vi "Pre-Bury Hook.vi"(8 "Error In":errorcluster) -> (0 "Error Out":errorcluster)   [LabVIEW 2018, in "Tests.lvlib" / "Toolkit.lvlib" / "Integration.lvlib"]
uses:
  Integration.lvlib
  Support/Bury Target.vi
  src/Toolkit/Toolkit.lvlib
  <vilib>/addons/_JKI Toolkits/Caraya/classes/Test/Test.lvclass
  Tests.lvlib
  <vilib>/addons/_JKI Toolkits/Caraya/classes/Assert/Assert.lvclass
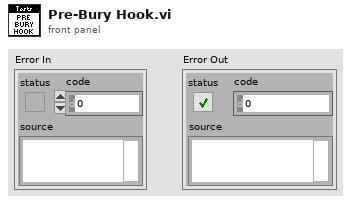
[diagram p1: front panel]
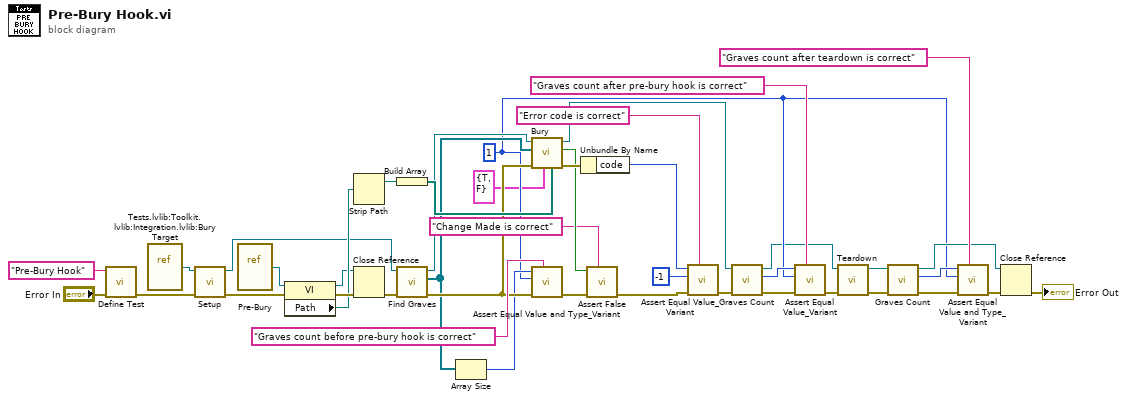
[diagram p0: block diagram]
diagram:
  w8 = 1 ("size(s)")
  n1 = call <vilib>:"Define Test.vi"("error in (no error)"="Error In", "Label (VI Title)"="Pre-Bury Hook") -> ("error out"=w38:errorcluster)  [unwired: 9 in]
  n2 = vi-ref "Tests.lvlib:Toolkit.lvlib:Integration.lvlib:Bury Target.vi"() -> (w20:refnum<vi>)
  n3 = call "Setup.vi"("Error In"=w38, "VI In"=w20) -> ("Error Out"=w28:errorcluster, "VI Out"=w17:refnum<vi>)  [unwired: 8 in]
  n4 = vi-ref "Pre-Bury.vi"() -> (w19:refnum<vi>)
  n5 = property class="VI"(reference=w19, error in=w28) -> (reference out=w24:refnum<vi>, error out=w27:errorcluster, "Path"=w26:path)
  n6 = Strip Path(path=w26) -> (stripped path=w25:path)  [unwired: 1 out]
  n7 = Close Reference(reference=w24, error in (no error)=w27) -> (error out=w18:errorcluster)
  n8 = Build Array(w25) -> (w21:path[])
  n9 = call "Find Graves.vi"("Error In"=w18, "VI In"=w17) -> ("Error Out"=w15:errorcluster, "Graves"=w14:refnum<vi>[], "VI Out"=w16:refnum<vi>)  [unwired: 7 in]
  n10 = Array Size(array=w14) -> (size(s)=w13:i32)
  n11 = call "Bury.vi"("Hook Search Path"=w21, "Execute Hooks?"=cluster{"Pre":bool, "Post":bool} {"Pre"=TRUE, "Post"=FALSE}, "Error In"=w15, "Graves"=w14, "VI In"=w16) -> ("Error Out"=w12:errorcluster, "Change Made?"=w2:bool, "VI Out"=w6:refnum<vi>)  [unwired: 4 in]
  n12 = call <vilib>:"Assert Equal Value and Type_Variant.vi"("Label"="Graves count before pre-bury hook is correct", "error in (no error)"=w15, "Y"=w8, "X"=w13) -> ("error out"=w37:errorcluster)  [unwired: 7 in]
  n13 = Unbundle By Name(w12) -> ("code"=w23:i32)
  n14 = call <vilib>:"Assert False.vi"("Label"="Change Made is correct", "error in (no error)"=w37, "False?"=w2) -> ("error out"=w3:errorcluster)  [unwired: 8 in]
  n15 = call <vilib>:"Assert Equal Value_Variant.vi"("Label"="Error code is correct", "error in (no error)"=w3, "Y"=-1 ("code"), "X"=w23) -> ("error out"=w11:errorcluster)  [unwired: 7 in]
  n16 = call "Graves Count.vi"("Error In"=w11, "Test Target In"=w6) -> ("Error Out"=w10:errorcluster, "Graves Count"=w9:i32, "Test Target Out"=w7:refnum<vi>)  [unwired: 7 in]
  n17 = call <vilib>:"Assert Equal Value_Variant.vi"("Label"="Graves count after pre-bury hook is correct", "error in (no error)"=w10, "Y"=w8, "X"=w9) -> ("error out"=w5:errorcluster)  [unwired: 7 in]
  n18 = call "Teardown.vi"("Error In"=w5, "VI In"=w7) -> ("Error Out"=w31:errorcluster, "VI Out"=w33:refnum<vi>)  [unwired: 8 in]
  n19 = call "Graves Count.vi"("Error In"=w31, "Test Target In"=w33) -> ("Error Out"=w30:errorcluster, "Graves Count"=w29:i32, "Test Target Out"=w32:refnum<vi>)  [unwired: 7 in]
  n20 = call <vilib>:"Assert Equal Value and Type_Variant.vi"("Label"="Graves count after teardown is correct", "error in (no error)"=w30, "Y"=w8, "X"=w29) -> ("error out"=w35:errorcluster)  [unwired: 7 in]
  n21 = Close Reference(reference=w32, error in (no error)=w35) -> (error out=→"Error Out":errorcluster)
